vi "check_detect_code.vi"() -> ()   [LabVIEW 2019]
uses:
  <vilib>/Analysis/NI_AALPro.lvlib
  <vilib>/Analysis/_algsub.llb/Test Real Matrix Type.vi
  <vilib>/Analysis/_algsub.llb/Matrix Type for Test.ctl
  <vilib>/Analysis/7linalg.llb/Real Cholesky Factorization.vi
  <vilib>/Analysis/7linalg.llb/Real LU Factorization.vi
  <vilib>/Analysis/7linalg.llb/Real QR Decomposition.vi
  <vilib>/Rock Robotics/WPI/ThirdParty/JAS_Junk/TrajLib/Trajectory_Library.lvlib
  <vilib>/Analysis/NI_AALBase.lvlib
  <vilib>/Analysis/baseanly.llb/Real A x B.vi
  <vilib>/Analysis/Matrix/Datatypes/RealMatrix.ctl
  <vilib>/Analysis/Matrix/NI_Matrix.lvlib
panel:
  out "error out":errorcluster
  out "LDLT Q":T1
  out "LDLT C":T1
  out "Pos Semi Definite":bool
  out "C":T1
  out "Q_Check":T1
  out "Bad":bool
  out "Stable Bad":bool
  out "Q_Chk_Passed":bool
  in  "A":T1
  out "D":T1
  out "L 2":T1
  out "QR error":i32
  out "R":T1
  out "Q":T1
  out "LU Error":i32
  out "U":T1
  out "L":T1
  out "Chol Error":i32
  out "Cholesky":T1
  out "symetric":bool
  out "pos semi definite":bool
  out "pos definite":bool
  in  "Real Matrix 2":T1
  in  "Q Input":T1
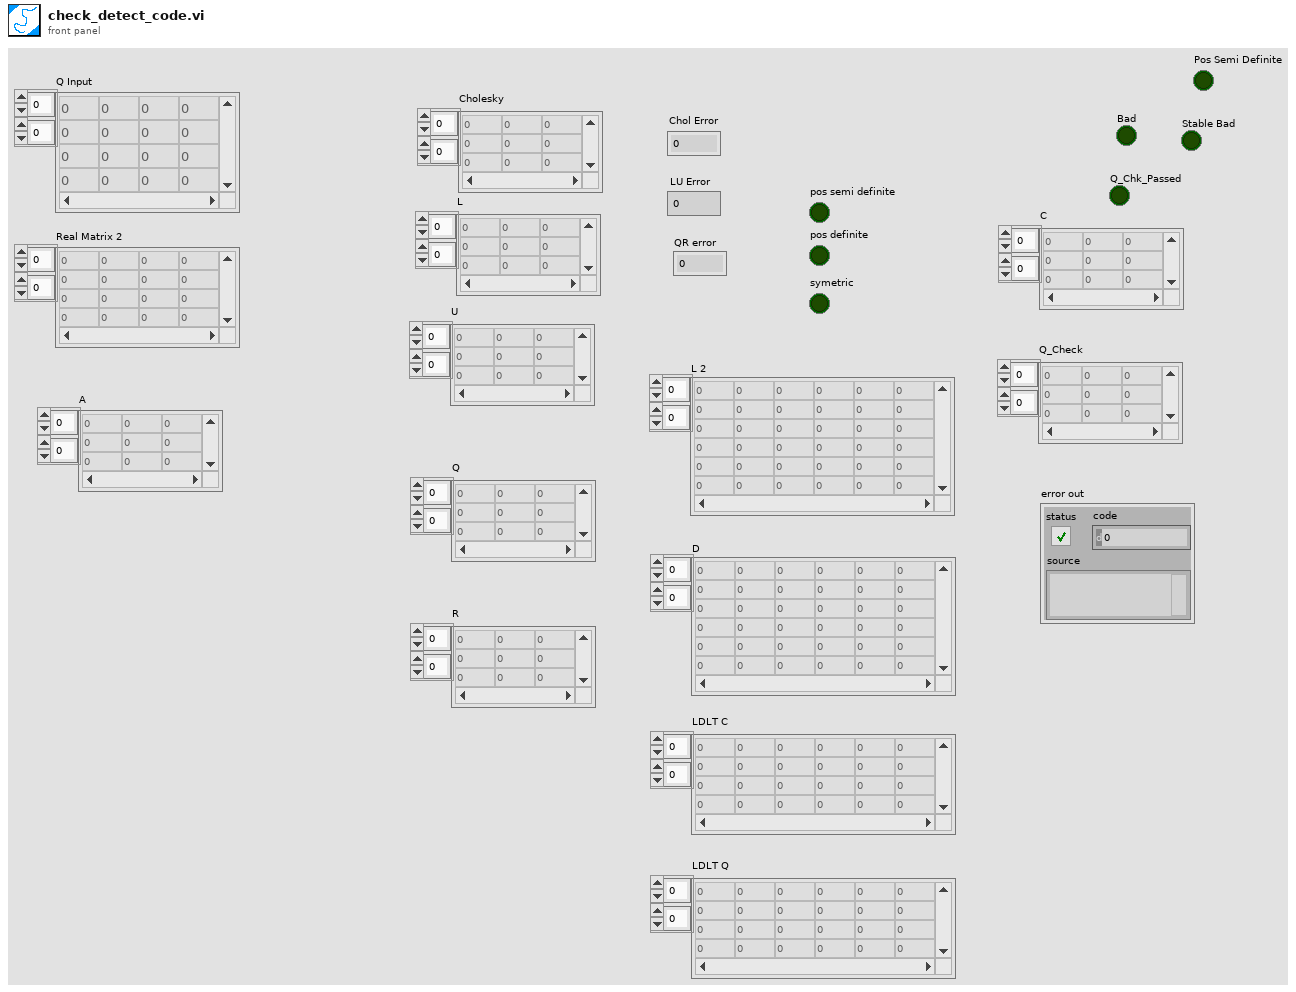
[diagram p1: front panel]
types:
  T1 = typedef "NI_Matrix.lvlib/RealMatrix.ctl" = dbl[][]
  T2 = typedef "NI_AALPro.lvlib/Matrix Type for Test.ctl" = i32
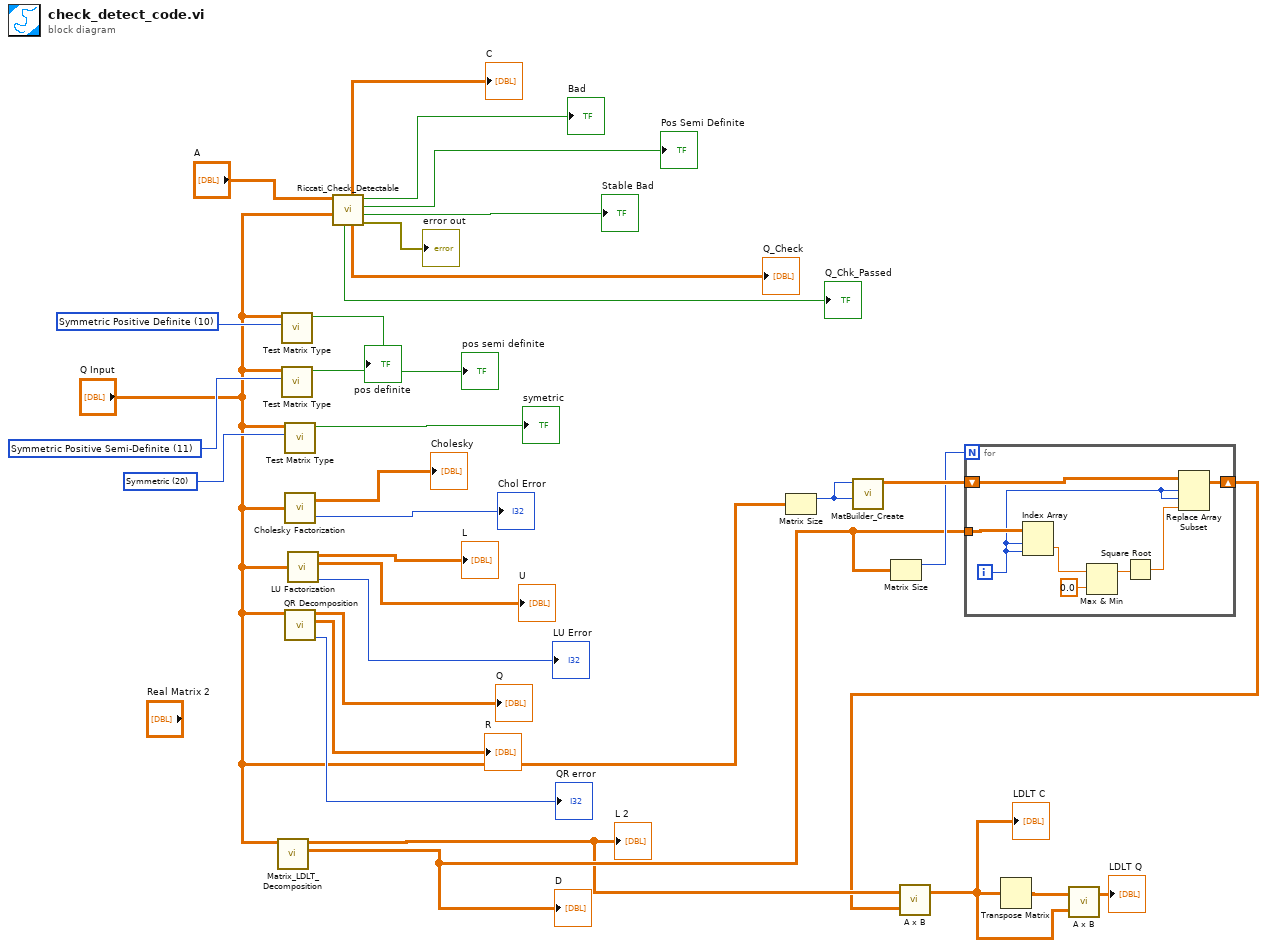
[diagram p0: block diagram]
diagram:
  w30 = T2 20 items=["Symmetric Positive Definite"=10, "Symmetric Positive Semi-Definite"=11, "Symmetric"=20, "Hermitian"=21] ("matrix type")
  w31 = T2 11 items=["Symmetric Positive Definite"=10, "Symmetric Positive Semi-Definite"=11, "Symmetric"=20, "Hermitian"=21] ("matrix type")
  w32 = T2 10 items=["Symmetric Positive Definite"=10, "Symmetric Positive Semi-Definite"=11, "Symmetric"=20, "Hermitian"=21] ("matrix type")
  n1 = call <vilib>:"Matrix_LDLT_Decomposition.vi"("Input Matrix"="Q Input") -> ("D"=w11:T1, "L"=w10:T1)  [unwired: 9 in]
  "L 2" <- w10
  "D" <- w11
  n2 = call-poly <vilib>:"Test Matrix Type.vi"("matrix type"=w32, "Input Matrix"="Q Input") -> ("is type?"=→"pos definite":bool)  [unwired: 8 in, 1 out]
  n3 = call-poly <vilib>:"Test Matrix Type.vi"("matrix type"=w31, "Input Matrix"="Q Input") -> ("is type?"=→"pos semi definite":bool)  [unwired: 8 in, 1 out]
  n4 = call-poly <vilib>:"Test Matrix Type.vi"("matrix type"=w30, "Input Matrix"="Q Input") -> ("is type?"=→"symetric":bool)  [unwired: 8 in, 1 out]
  n5 = call-poly <vilib>:"Cholesky Factorization.vi"("A"="Q Input") -> ("Cholesky"=→"Cholesky":T1, "error"=→"Chol Error":i32)
  n6 = call-poly <vilib>:"QR Decomposition.vi"("A"="Q Input") -> ("error"=→"QR error":i32, "R"=→"R":T1, "Q"=→"Q":T1)  [unwired: 7 in, 1 out]
  n7 = call-poly <vilib>:"LU Factorization.vi"("A"="Q Input") -> ("L"=→"L":T1, "U"=→"U":T1, "error"=→"LU Error":i32)  [unwired: 1 out]
  n8 = call <vilib>:"Riccati_Check_Detectable.vi"("Q"="Q Input", "A"="A") -> ("error out"=→"error out":errorcluster, "Stable Bad"=→"Stable Bad":bool, "Pos Semi Definite"=→"Pos Semi Definite":bool, "Bad"=→"Bad":bool, "Q_Check"=→"Q_Check":T1, "C"=→"C":T1, "Q_Chk_Passed"=→"Q_Chk_Passed":bool)  [unwired: 3 in]
  n9 = Matrix Size(0:"Q Input") -> (1:w15:i32)  [unwired: 1 out]
  n10 = call <vilib>:"MatBuilder_Create.vi"("Columns"=w15, "Rows"=w15) -> ("output matrix"=w14:T1)  [unwired: 9 in]
  n11 = Matrix Size(0:w11) -> (1:w13:i32)  [unwired: 1 out]
  n12 = for {
    N: w13 -> [_]
    tunnel: w11 -> [w40]
    shift-right: [w38] -> w9
    shift-left: w14 -> [w39]
    i -> [w33]
    n13 = Index Array(array=w40, index (row)=w33, index (col)=w33) -> (element=w36:dbl)
    n14 = Max & Min(x=w36, y=0.0) -> (max(x,y)=w34:dbl)  [unwired: 1 out]
    n15 = Square Root ("Square Root.vi")(x=w34) -> (sqrt(x)=w37:dbl)
    n16 = Replace Array Subset(array=w39, new element=w37, index (row)=w33, index (col)=w33) -> (w38:T1)
  }
  n17 = call-poly <vilib>:"A x B.vi"("B"=w9, "A"=w10) -> ("A x B"=w7:T1)  [unwired: 1 out]
  "LDLT C" <- w7
  n18 = Transpose Matrix(1:w7) -> (0:w8:T1)
  n19 = call-poly <vilib>:"A x B.vi"("B"=w7, "A"=w8) -> ("A x B"=→"LDLT Q":T1)  [unwired: 1 out]
